vi "Sensor Distance Capture.vi"(9 "X":dbl) -> (2 "Y":dbl)   [LabVIEW 2016]
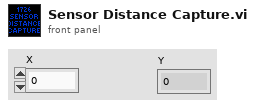
[diagram p1: front panel]
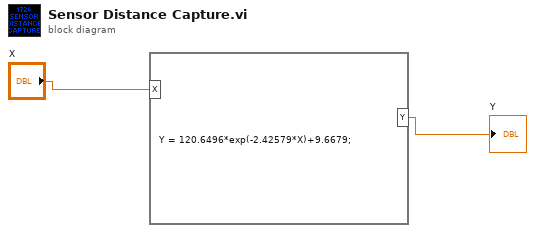
[diagram p0: block diagram]
diagram:
  n1 = formula code="Y = 120.6496*exp(-2.42579*X)+9.6679;"("X"="X") -> ("Y"=→"Y":dbl)
